vi "Repeated start.vi"(9 "Min time SCL low (uSec)":u32 caption="Min time SCL low  (uSec)", 10 "Min time SCL high (uSec)":u32) -> ()   [LabVIEW 2013]
uses:
  <vilib>/rvi/eio/common/nirviEmuTemplateMethod_errors.vi
  <vilib>/eio/EIONode/EIONode.xnode
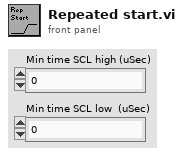
[diagram p1: front panel]
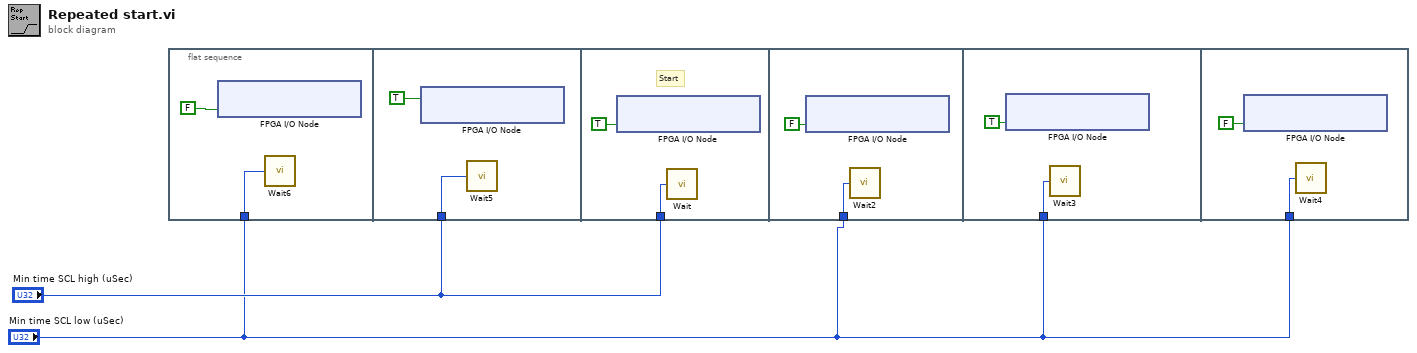
[diagram p0: block diagram]
diagram:
  n1 = flat-sequence {
    tunnel: "Min time SCL low (uSec)" -> [w3]
    tunnel: "Min time SCL high (uSec)" -> [w5]
    tunnel: "Min time SCL high (uSec)" -> [w7]
    tunnel: "Min time SCL low (uSec)" -> [w9]
    tunnel: "Min time SCL low (uSec)" -> [w11]
    tunnel: "Min time SCL low (uSec)" -> [w13]
    frame #0 {
      n2 = xnode "FPGA I/O Node"("ConnectorB/DIO13"=FALSE ("ConnectorC/DIO1")) -> ()  [unwired: 1 in, 1 out]
      n3 = call "Wait6"("Count(uSec)"=w3) -> ()  [unwired: 1 out]
    }
    frame #1 {
      n4 = xnode "FPGA I/O Node"("ConnectorB/DIO12"=TRUE ("ConnectorC/DIO0")) -> ()  [unwired: 1 in, 1 out]
      n5 = call "Wait5"("Count(uSec)"=w5) -> ()  [unwired: 1 out]
    }
    frame #2 {
      # "Start"
      n6 = xnode "FPGA I/O Node"("ConnectorB/DIO13"=TRUE ("ConnectorC/DIO0")) -> ()  [unwired: 1 in, 1 out]
      n7 = call "Wait"("Count(uSec)"=w7) -> ()  [unwired: 1 out]
    }
    frame #3 {
      n8 = xnode "FPGA I/O Node"("ConnectorB/DIO12"=FALSE ("ConnectorC/DIO1")) -> ()  [unwired: 1 in, 1 out]
      n9 = call "Wait2"("Count(uSec)"=w9) -> ()  [unwired: 1 out]
    }
    frame #4 {
      n10 = xnode "FPGA I/O Node"("ConnectorB/DIO12"=TRUE ("ConnectorC/DIO1")) -> ()  [unwired: 1 in, 1 out]
      n11 = call "Wait3"("Count(uSec)"=w11) -> ()  [unwired: 1 out]
    }
    frame #5 {
      n12 = xnode "FPGA I/O Node"("ConnectorB/DIO13"=FALSE ("ConnectorC/DIO0")) -> ()  [unwired: 1 in, 1 out]
      n13 = call "Wait4"("Count(uSec)"=w13) -> ()  [unwired: 1 out]
    }
  }
